vi "Dictionary Path--constant.vi"() -> (3 "appended path":path)   [LabVIEW 2024, in "Application.lvlib"]
uses:
  Application.lvlib
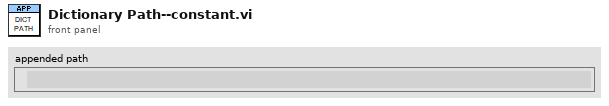
[diagram p1: front panel]
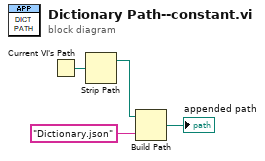
[diagram p0: block diagram]
diagram:
  n1 = Current VI's Path() -> (path=w1:path)
  n2 = Strip Path(path=w1) -> (stripped path=w2:path)  [unwired: 1 out]
  n3 = Build Path(base path=w2, name or relative path="Dictionary.json") -> (appended path=→"appended path":path)
